vi "Update Fan State.vi"(8 "error in":errorcluster, 11 "tCRD in":refnum<class "Aircraft OPCCRD.lvclass">) -> (0 "error out":errorcluster, 3 "tCRD out":refnum<class "Aircraft OPCCRD.lvclass">)   [LabVIEW 2015, in "Aircraft OPCCRD.lvclass"]
uses:
  Aircraft OPCCRD.lvclass
  <vilib>/rvi/interface/nirviReadWriteControl/nirviReadWriteControl.xnode
  tFPGA Ref.ctl
  NiFpgaLv.dll
  <vilib>/Utility/error.llb/Error Cluster From Error Code.vi
  <vilib>/rvi/errors/niLvFpgaAdjustHostInterfaceError.vi
  Reusable/Session Log/System Log.lvclass
  FPGA Bitfiles/FPGAServerwLRS.lvbitx
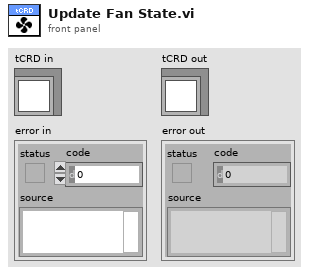
[diagram p1: front panel]
types:
  T1 = typedef "Session - Root.lvclass/Session Handle.ctl" = refnum<data-value>
  T2 = typedef "tCRD.lvclass/tFPGA Ref.ctl" = refnum<k20>
  T3 = typedef "Aircraft OPCCRD.lvclass/tFPGA Ref.ctl" = refnum<k20>
  T4 = cluster{"Bank 1":bool, "Bank 2":bool, "Bank 3":bool}
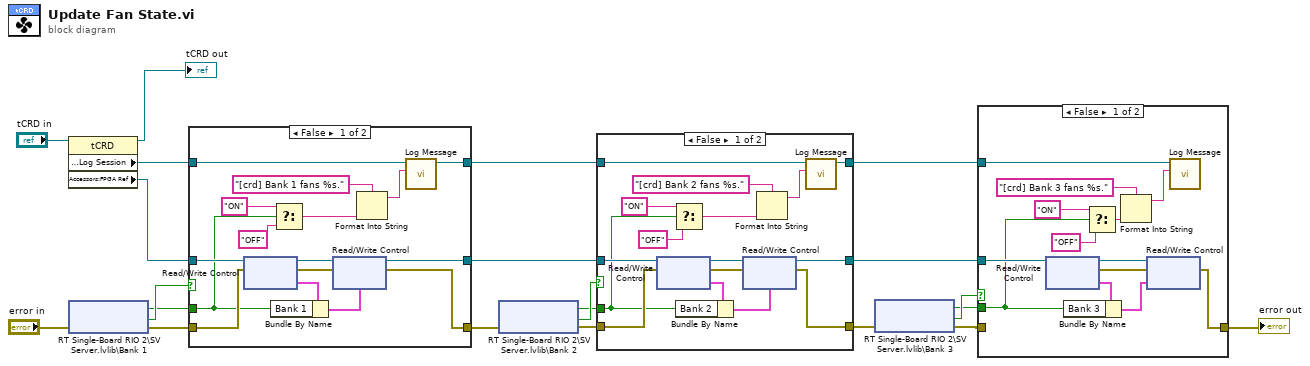
[diagram p0: block diagram]
diagram:
  n1 = property class="tCRD"(reference="tCRD in") -> (reference out=→"tCRD out":refnum<class "Aircraft OPCCRD.lvclass">, "Accessors:Log Session"=w4:T1, "Accessors:FPGA Ref"=w5:T2)  [unwired: 1 in, 1 out]
  n2 = shared-variable "RT Single-Board RIO 2\\SV Server.lvlib\\Bank 1"(error in="error in") -> (w9:bool, error out=w17:errorcluster, w21:bool)  [unwired: 1 in]
  n3 = case shown="False" w21 {
    tunnel: w5 -> [w36 w40]
    tunnel: [w37 w40] -> w19
    tunnel: w17 -> [w31 w39]
    tunnel: [w30 w39] -> w16
    tunnel: w9 -> [w26 _]
    tunnel: w4 -> [w29 w38]
    tunnel: [w22 w38] -> w3
    frame False {
      n4 = xnode "Read/Write Control"("FPGA VI Reference In"=w36, "error in"=w31) -> ("FPGA VI Reference Out"=w33:T3, "error out"=w32:errorcluster, "Fans"=w35:T4)
      n5 = Bundle By Name(cluster=w35, "Bank 1"=w26) -> (w34:T4)
      n6 = Select(t="ON", s=w26, f="OFF") -> (s? t:f=w24:string)
      n7 = xnode "Read/Write Control"("FPGA VI Reference In"=w33, "error in"=w32, "Fans"=w34) -> ("FPGA VI Reference Out"=w37:T3, "error out"=w30:errorcluster)
      n8 = Format Into String(format string="[crd] Bank 1 fans %s." ("MSG In"), w24) -> (resulting string=w23:string)  [unwired: 2 in, 1 out]
      n9 = call "Log Message.vi"("MSG In"=w23, "session in"=w29) -> ("session out"=w22:T1)  [unwired: 8 in, 1 out]
    }
    frame True {
    }
  }
  n10 = shared-variable "RT Single-Board RIO 2\\SV Server.lvlib\\Bank 2"(error in=w16) -> (w10:bool, error out=w15:errorcluster, w18:bool)  [unwired: 1 in]
  n11 = case shown="False" w18 {
    tunnel: w19 -> [w52 w59]
    tunnel: [w50 w59] -> w11
    tunnel: w15 -> [w51 w58]
    tunnel: [w49 w58] -> w14
    tunnel: w10 -> [w43 _]
    tunnel: w3 -> [w44 w57]
    tunnel: [w42 w57] -> w1
    frame False {
      n12 = xnode "Read/Write Control"("FPGA VI Reference In"=w52, "error in"=w51) -> ("FPGA VI Reference Out"=w54:T3, "error out"=w53:errorcluster, "Fans"=w56:T4)
      n13 = Select(t="ON", s=w43, f="OFF") -> (s? t:f=w47:string)
      n14 = Bundle By Name(cluster=w56, "Bank 2"=w43) -> (w55:T4)
      n15 = xnode "Read/Write Control"("FPGA VI Reference In"=w54, "error in"=w53, "Fans"=w55) -> ("FPGA VI Reference Out"=w50:T3, "error out"=w49:errorcluster)
      n16 = Format Into String(format string="[crd] Bank 2 fans %s." ("MSG In"), w47) -> (resulting string=w48:string)  [unwired: 2 in, 1 out]
      n17 = call "Log Message.vi"("MSG In"=w48, "session in"=w44) -> ("session out"=w42:T1)  [unwired: 8 in, 1 out]
    }
    frame True {
    }
  }
  n18 = shared-variable "RT Single-Board RIO 2\\SV Server.lvlib\\Bank 3"(error in=w14) -> (w7:bool, error out=w13:errorcluster, w12:bool)  [unwired: 1 in]
  n19 = case shown="False" w12 {
    tunnel: w11 -> [w68 _]
    tunnel: w13 -> [_ w73]
    tunnel: [w67 w73] -> w8
    tunnel: w7 -> [w62 _]
    tunnel: w1 -> [w61 _]
    frame False {
      n20 = xnode "Read/Write Control"("FPGA VI Reference In"=w68) -> ("FPGA VI Reference Out"=w70:T3, "error out"=w69:errorcluster, "Fans"=w72:T4)  [unwired: 1 in]
      n21 = Bundle By Name(cluster=w72, "Bank 3"=w62) -> (w71:T4)
      n22 = Select(t="ON", s=w62, f="OFF") -> (s? t:f=w64:string)
      n23 = Format Into String(format string="[crd] Bank 3 fans %s." ("MSG In"), w64) -> (resulting string=w63:string)  [unwired: 2 in, 1 out]
      n24 = xnode "Read/Write Control"("FPGA VI Reference In"=w70, "error in"=w69, "Fans"=w71) -> ("error out"=w67:errorcluster)  [unwired: 1 out]
      n25 = call "Log Message.vi"("MSG In"=w63, "session in"=w61) -> ()  [unwired: 8 in, 2 out]
    }
    frame True {
    }
  }
  "error out" <- w8
